vi "Initialize.vi"(6 "called by VI":string, 8 "error in (no error)":errorcluster, 9 "create if not found? (T)":bool=TRUE, 10 "name (unnamed)":string, 11 "Object in":refnum<class "OpenG_Reference_Object.lvclass">) -> (0 "error out":errorcluster, 1 "created new?":bool, 3 "Object out":refnum<class "OpenG_Reference_Object.lvclass">)   [LabVIEW 2015, in "OpenG_Reference_Object.lvclass"]
doc: "Initializes object data containers."
uses:
  <userlib>/_OpenG.lib/openg_object/openg_reference_object.llb/OpenG_Reference_Object.lvclass
  <userlib>/_OpenG.lib/openg_object/openg_reference_object.llb/Key.ctl
  <userlib>/_OpenG.lib/openg_object/openg_reference_object.llb/OpenG_Reference_Object.lvclass/OpenG_Reference_Object.ctl
  <userlib>/_OpenG.lib/openg_object/openg_reference_object.llb/DebuggerModes.ctl
  <userlib>/_OpenG.lib/openg_object/openg_object.llb/OpenG_Object.lvclass
panel:
  # "Please visit http://www.OpenG.org to learn about the\nOpen Source LabVIEW software movement.\n\nNOTICE -- YOU MUST LEAVE THIS NOTICE IN PLACE.  PER THE TERMS OF THE LICENSE BELOW, YOU MAY SUBLICENSE THIS SOFTWARE \nIN ANY WAY THAT DOES NOT CONFLICT WITH THIS LICENSE.\n\n### BSD License (http://www.opensource.org/licenses/bsd-license.php) Begin ###\n\nCopyright (c) 2007, Tomi Maila\nCopyright (c) 2007, Endevo AB\n\n\nAll rights reserved.\n\nRedistribution and use in source and binary forms, with or without modification, are permitted provided that the following conditions are met:\n\n    * Redistributions of source code must retain the above copyright notice, this list of conditions and the following disclaimer.\n    * Redistributions in binary form must reproduce the above copyright notice, this list of conditions and the following disclaimer in the \n       documentation and/or other materials provided with the distribution.\n    * Neither the name of Endevo AB nor the names of the contributors may be used to endorse or promote products derived\n       from this software without specific prior written permission.\n\nTHIS SOFTWARE IS PROVIDED BY THE COPYRIGHT HOLDERS AND CONTRIBUTORS \"AS IS\" AND ANY EXPRESS OR IMPLIED WARRANTIES, \nINCLUDING, BUT NOT LIMITED TO, THE IMPLIED WARRANTIES OF MERCHANTABILITY AND FITNESS FOR A PARTICULAR PURPOSE ARE \nDISCLAIMED. IN NO EVENT SHALL THE COPYRIGHT OWNER OR CONTRIBUTORS BE LIABLE FOR ANY DIRECT, INDIRECT, INCIDENTAL,\n SPECIAL, EXEMPLARY, OR CONSEQUENTIAL DAMAGES (INCLUDING, BUT NOT LIMITED TO, PROCUREMENT OF SUBSTITUTE GOODS OR \nSERVICES; LOSS OF USE, DATA, OR PROFITS; OR BUSINESS INTERRUPTION) HOWEVER CAUSED AND ON ANY THEORY OF LIABILITY, \nWHETHER IN CONTRACT, STRICT LIABILITY, OR TORT (INCLUDING NEGLIGENCE OR OTHERWISE) ARISING IN ANY WAY OUT OF THE USE \nOF THIS SOFTWARE, EVEN IF ADVISED OF THE POSSIBILITY OF SUCH DAMAGE.\n\n### BSD License End ###"
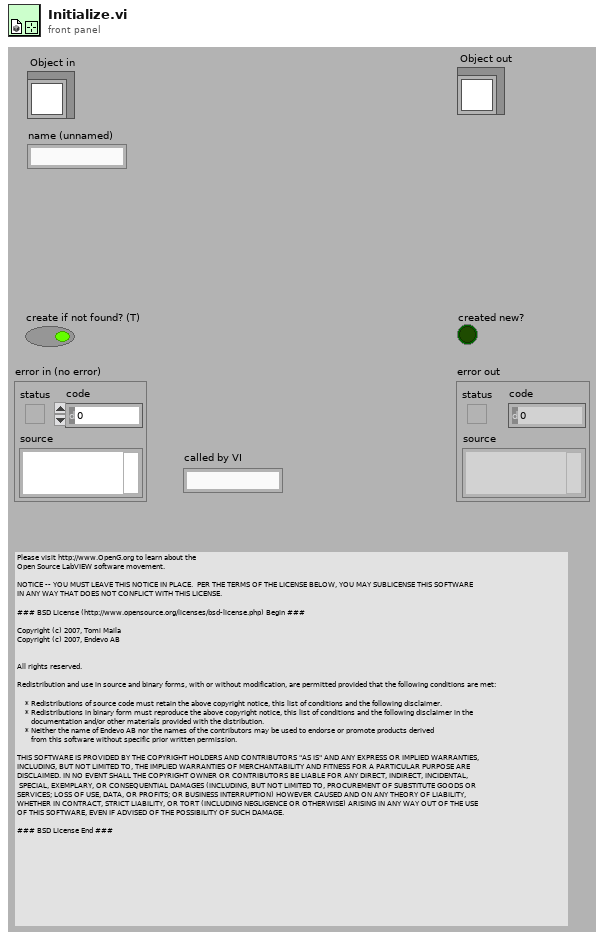
[diagram p1: front panel]
types:
  T1 = typedef "OpenG_Reference_Object.lvclass/Key.ctl" = refnum<k1>
  T2 = typedef "OpenG_Reference_Object.lvclass/DebuggerModes.ctl" = enum16{"insert", "remove", "preview", "clear", "remove invalid"}
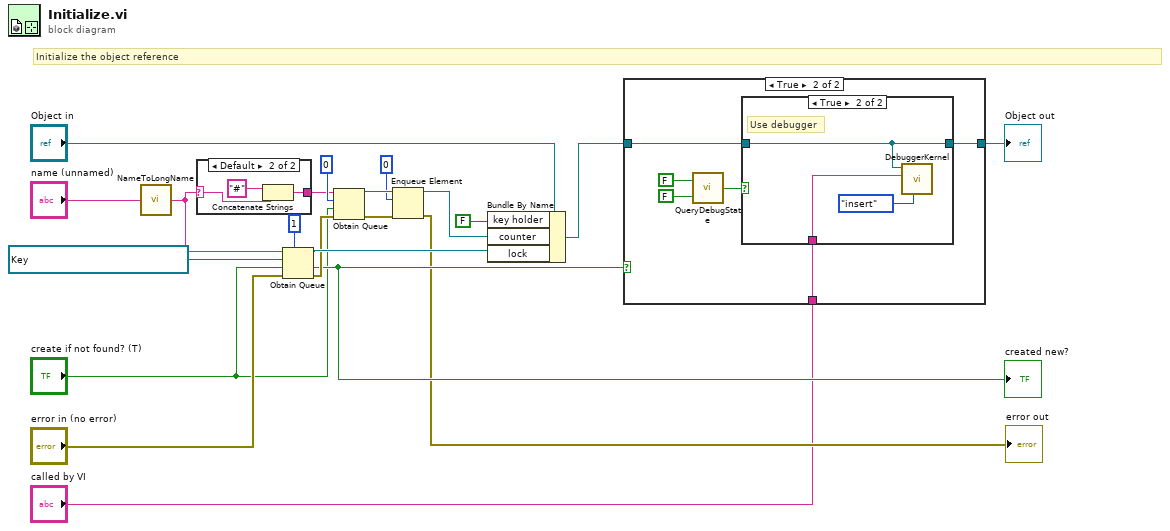
[diagram p0: block diagram]
diagram:
  w16 = T1 refnum items=["Open Reference Object Key"] ("Open Reference Object Key")
  # "Initialize the object reference"
  n1 = call <userlib>:"NameToLongName.vi"("name in"="name (unnamed)") -> ("long name out"=w7:string)
  n2 = case shown="Default" w7 {
    selector: w7 -> [w22 w23]
    tunnel: [w22 w25] -> w8
    frame "" {
    }
    frame Default {
      n3 = Concatenate Strings("#" ("string"), w23) -> (w25:string)
    }
  }
  n4 = Obtain Queue(max queue size (-1, unlimited)=1, name (unnamed)=w7, element data type=w16, create if not found? (T)="create if not found? (T)", error in (no error)="error in (no error)") -> (queue out=w17:refnum<queue>, created new?=w6:bool, error out=w10:errorcluster)
  "created new?" <- w6
  n5 = Obtain Queue(name (unnamed)=w8, element data type=u8 0, create if not found? (T)="create if not found? (T)", error in (no error)=w10) -> (queue out=w14:refnum<queue>, error out=w15:errorcluster)  [unwired: 1 in, 1 out]
  n6 = Enqueue Element(queue=w14, element=u8 0, error in (no error)=w15) -> (queue out=w11:refnum<queue>, error out=→"error out":errorcluster)  [unwired: 1 in, 1 out]
  n7 = Bundle By Name(cluster="Object in", "key holder"=FALSE ("lock owner"), "counter"=w11, "lock"=w17) -> (w5:refnum<class "OpenG_Reference_Object.lvclass">)
  n8 = case shown="True" w6 {
    tunnel: w5 -> [w26 w29]
    tunnel: [w26 w28] -> w4
    tunnel: "called by VI" -> [_ w27]
    frame False {
    }
    frame True {
      n9 = call <userlib>:"QueryDebugState.vi"("set to state (F)"=FALSE, "set? (F)"=FALSE) -> ("debug?"=w30:bool)
      n10 = case shown="True" w30 {
        tunnel: w29 -> [w33 w36]
        tunnel: [w33 w36] -> w28
        tunnel: w27 -> [_ w34]
        frame False {
        }
        frame True {
          # "Use debugger"
          n11 = call <userlib>:"DebuggerKernel.vi"("Mode"=DebuggerModes."insert", "Created in VI"=w34, "Object in"=w36) -> ()  [unwired: 8 in, 1 out]
        }
      }
    }
  }
  "Object out" <- w4
